vi "Gel Tugging Force Mode_Data Reduction v16.00.vi"() -> ()   [LabVIEW 2015]
doc: "I. Description:\nThis example demonstrates how to continuously acquire and generate data at the same time, synchronized with one another.\n\nII. Instructions for Running:\n1. Select the physical channel to correspond to where your signal is input on the DAQ device. Also, select the corresponding channel for where your signal is being generated.\n2. Enter the minimum and maximum voltage ranges.\nNote: For better accuracy try to match the input range to the expected voltage level of the measured signal.\n3. Set the sample rate of the acquisition.\nNote: The rate should be at least twice as fast as the maximum frequency component of the signal being acquired. \n6. Select the Rate for the generation\n7. Select what type of signal to generate and the amplitude.\nNote: This example requires two DMA channels to run. If your hardware does not support two DMA channels, you need to set the Data Transfer Mechanism property for the Analog Output Task to use \"Interrupts\". The Data Transfer Mechanism property is located in the DAQmx Channel Property hierarchy at:\n\nDAQmx Channel Property Node>>Analog Output>>General Properties>>Advanced>>Data Transfer and Memory>>Data Transfer Mechanism\n\nRefer to your device documentation to determine how many DMA channels are supported for your hardware.\n\nIII. Block Diagram Steps:\n1. Create an analog input voltage channel. Also, create an analog output voltage channel.\n2. Set the rate for the sample clock. Additionally, define the sample mode to be continuous. Also, set the sample clock rate for the signal generation.\n2a. Call the Get Terminal Name with Device Prefix VI. This will take a Task and a terminal and create a properly formatted device + terminal name to use as the source of the Trigger.\n3. Define the parameters for a Digital Edge Start Trigger. Set the Analog output to trigger off the AI Start Trigger. This is an internal trigger signal.\n4. Use the Basic Function Generator VI to create the signal to be generated.\n5. Call the Start VI to arm the two functions. Make sure the analog output is armed before the analog input. This will ensure both will start at the same time.\n6. Read the waveform data in a loop until the user hits the stop button or an error occurs. The Is Task Done? VI is used to check for errors in the Analog Output Task.\n7. Call the Clear VI to Clear the Task\n8. Use the popup dialog box to display an error if any.\n\nIV. I/O Connections Overview:\nMake sure your signal input/output terminals match the Physical Channel I/O controls."
uses:
  <vilib>/Utility/file.llb/Read Delimited Spreadsheet (DBL).vi
  <vilib>/Analysis/NI_AALBase.lvlib
  <vilib>/Analysis/NI_AALPro.lvlib
panel:
  out "Total Ramp\n Time (ms)":dbl format="%#_10g"
  out "# of Ramp\n Steps":dbl format="%#_10g"
  out "Fluoro Bead \nDiameter (um)":dbl format="%#_10g"
  out "Image Scale (Micron/Pixel)":dbl format="%#_10g"
  out "Initial Sep Distance (Micron)":dbl format="%#_10g"
  out "Fluoro Beads Z-Level (micron)":dbl format="%#_10g"
  out "Gel Thickness (micron)":dbl format="%#_10g"
  out "Magnetic Bead Z-Level (micron)":dbl format="%#_10g"
  out "Tip Z-Level (micron)":dbl format="%#_10g"
  out "Exposure \nPulses":i32
  out "Magnetic Bead Diameter (um)":dbl format="%#_10g"
  out "Null Flux\nCorrected (Gs)":dbl format="%#_10g"
  out "95% C.I. Maximum":dbl format="%_8f"
  out "95% C.I. Minimum":dbl format="%_8f"
  out "Current, Std Dev (V or Amp)":dbl format="%_8g"
  out "Current, Mean (V or Amp) 2":dbl format="%_8g"
  out "Slope of Trendline \n(mV of mAmp/min)":dbl
  out "Slope of Trendline \n(V or Amp/sec)":dbl
  out "Intercept of Trendline (V or Amp)":dbl format="%#_8g"
  out "Slope of Trendline \n(mV of mAmp/min)":dbl
  out "Intercept of Trendline (V or Amp)":dbl format="%#_8g"
  out "Slope of Trendline \n(V or Amp/sec)":dbl
  out "95% C.I. Maximum":dbl format="%_8f"
  out "95% C.I. Minimum":dbl format="%_8f"
  out "Current, Std Dev (V or Amp)":dbl format="%_8g"
  out "Current, Mean (V or Amp)":dbl format="%_8g"
  in  "Final Time 2 (s)":dbl=3.0 format="%_8g"
  in  "Initial Time 2 (s)":dbl=2.05 format="%_8g"
  out "Current Signal (V)":cluster{dbl[], dbl[]}(graph)
  out "Slope of Trendline \n(mGs/min)":dbl
  out "Intercept of Trendline (Gs)":dbl format="%#_8g"
  out "Slope of Trendline \n(Gs/sec)":dbl
  out "95% C.I. Maximum":dbl format="%_8f"
  out "95% C.I. Minimum":dbl format="%_8f"
  out "Magnetic Flux, Std Dev (Gs)":dbl format="%_8g"
  out "Magnetic Flux, Mean (Gs)":dbl format="%_8g"
  out "OFF PID gains":T1={"proportional gain (Kc)"=0.8, "integral time (Ti, min)"=3e-05, "derivative time (Td, min)"=4.7e-06} {"proportional gain (Kc)" format="%#_10g"; "integral time (Ti, min)" format="%#_10g"; "derivative time (Td, min)" format="%#_10g"}
  out "Relative Humidity (%)":dbl format="%#_10g"
  out "Needle Inclination Angle (º)":dbl format="%#_10g"
  out "Temperature (ºC)":dbl format="%#_10g"
  out "Post- Zero\nInterval (s) <(If not  interrupted)":dbl format="%#_10g"
  out "Pre- Zero \nInterval (s)":dbl format="%#_10g"
  out "Null Flux\nObserved (Gs)":dbl format="%#_10g"
  out "Flux ON Relative \nSetpoint (Gs)":dbl format="%#_10g"
  in  "Final Time 1 (s)":dbl=2.0 format="%_8g"
  in  "Initial Time 1 (s)":dbl=1.05 format="%_8g"
  out "PID Rate (Hz)":dbl format="%#_10g"
  out "Sampling Rate \n(Samples/Sec)":dbl format="%#_10g"
  out "ON PID gains":T1={"proportional gain (Kc)"=0.8, "integral time (Ti, min)"=3e-05, "derivative time (Td, min)"=4.7e-06} {"proportional gain (Kc)" format="%#_10g"; "integral time (Ti, min)" format="%#_10g"; "derivative time (Td, min)" format="%#_10g"}
  out "Samples Pushed \nto PID at a time":dbl format="%#_10g"
  out "Camera Exposure (V)":cluster{dbl[], dbl[]}(graph)
  out "# of Data Points":i32
  out "Sampling\nInterval (ms)":dbl format="%#_8g"
  out "Slope of Trendline \n(mGs/min)":dbl
  out "Intercept of Trendline (V)":dbl format="%#_8g"
  out "Slope of Trendline \n(Gs/sec)":dbl
  out "95% C.I. Maximum":dbl format="%_8f"
  out "95% C.I. Minimum":dbl format="%_8f"
  out "Magnetic Flux, Std Dev (Gs)":dbl format="%_8g"
  out "Magnetic Flux, Mean (Gs)":dbl format="%_8g"
  out "Magnetic Sensor \nSensitivity (V/Gs)":dbl
  out "Flux Signal, V":cluster{dbl[], dbl[]}(graph)
  out "Magnetic Sensor \nCalibrated Zero (V)":dbl format="%#_12g"
  out "Number of \nCycles":dbl format="%#_10g"
  out "Flux Signal, Gs":cluster{dbl[], dbl[]}(graph)
  in  "Select data file for reduction...":path
  # "Gel Testing v.15.00 + v15.10 + v15.20"
  # "Drift Analysis For Flux & Current:"
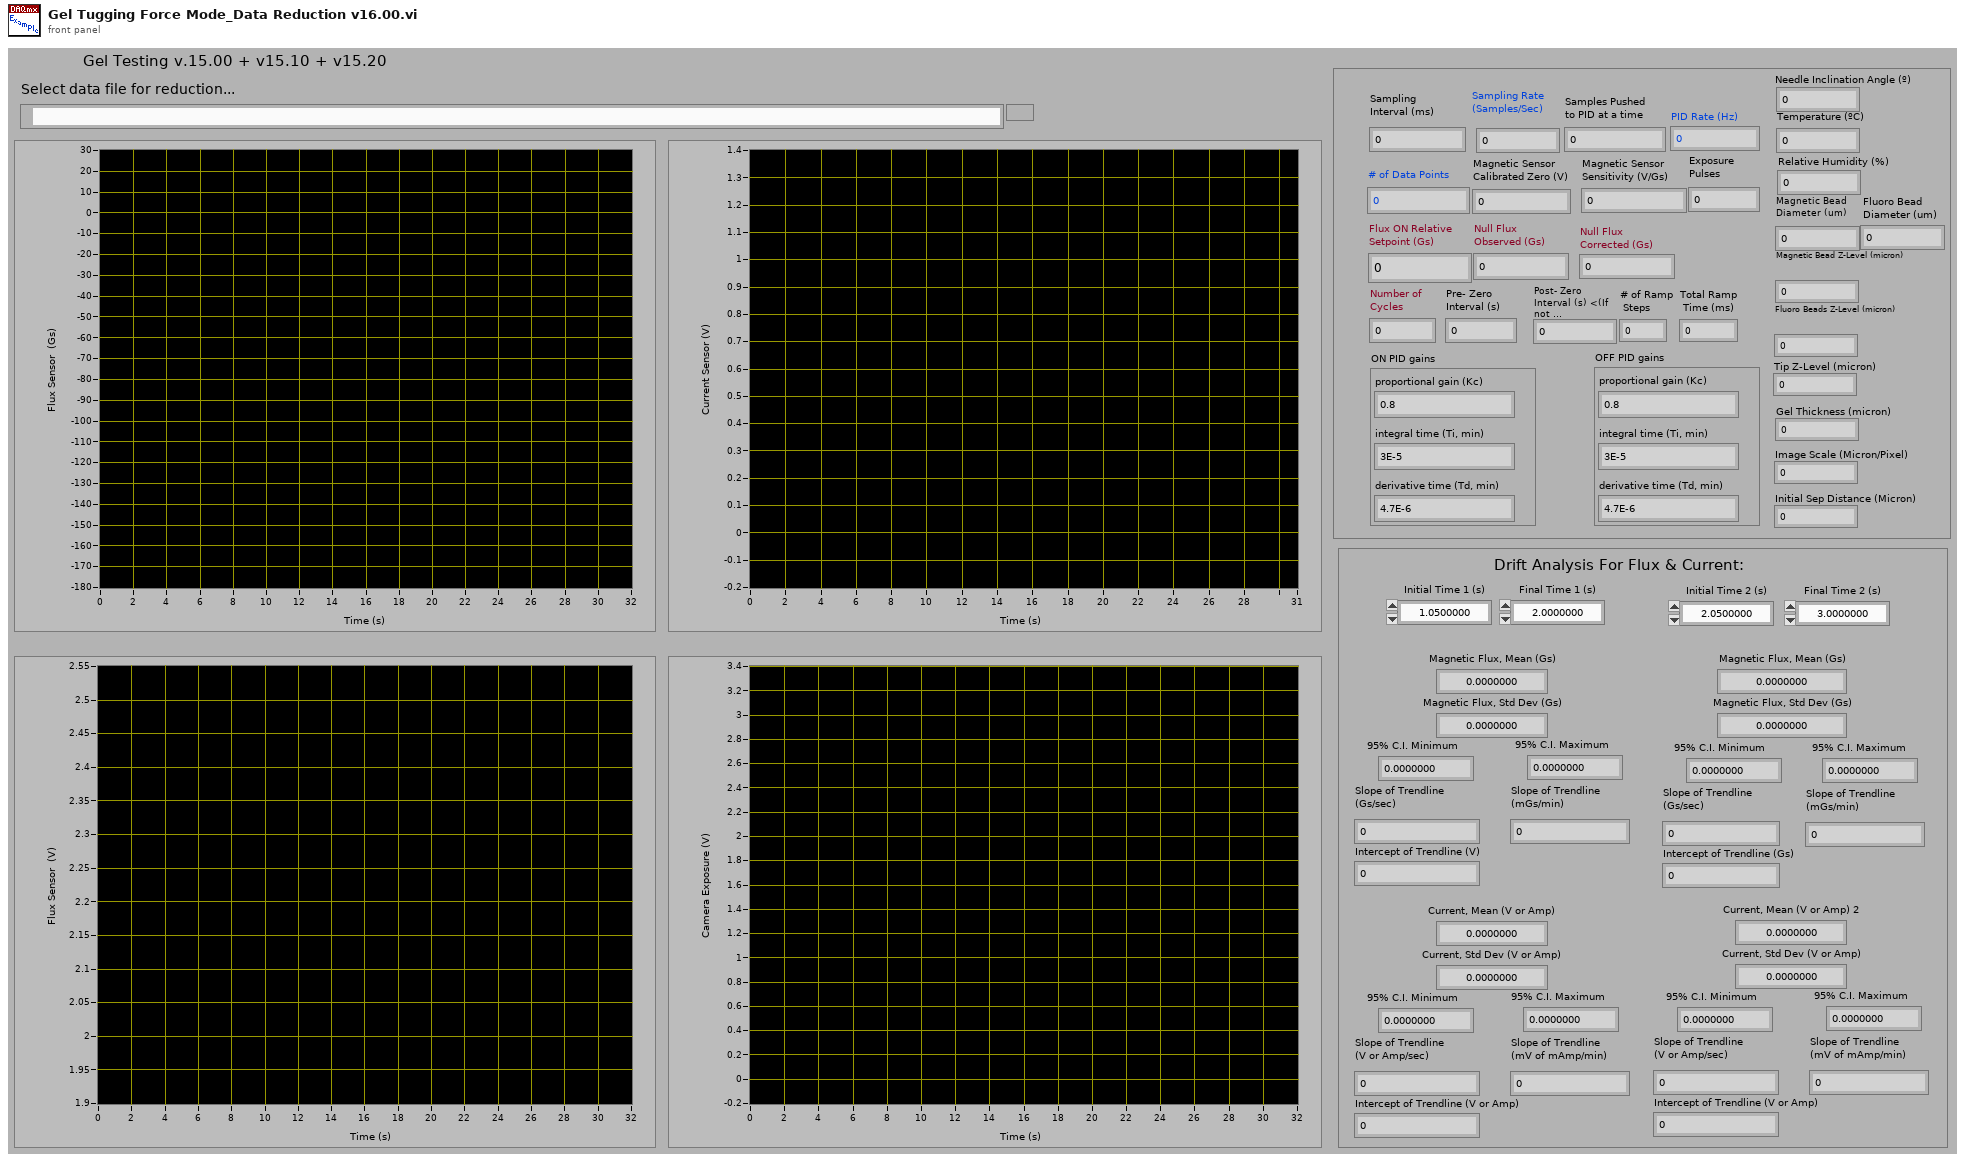
[diagram p1: front panel]
types:
  T1 = cluster{"proportional gain (Kc)":dbl, "integral time (Ti, min)":dbl, "derivative time (Td, min)":dbl}
  T2 = cluster{"Numeric":dbl, "Numeric":dbl, "Numeric":dbl}
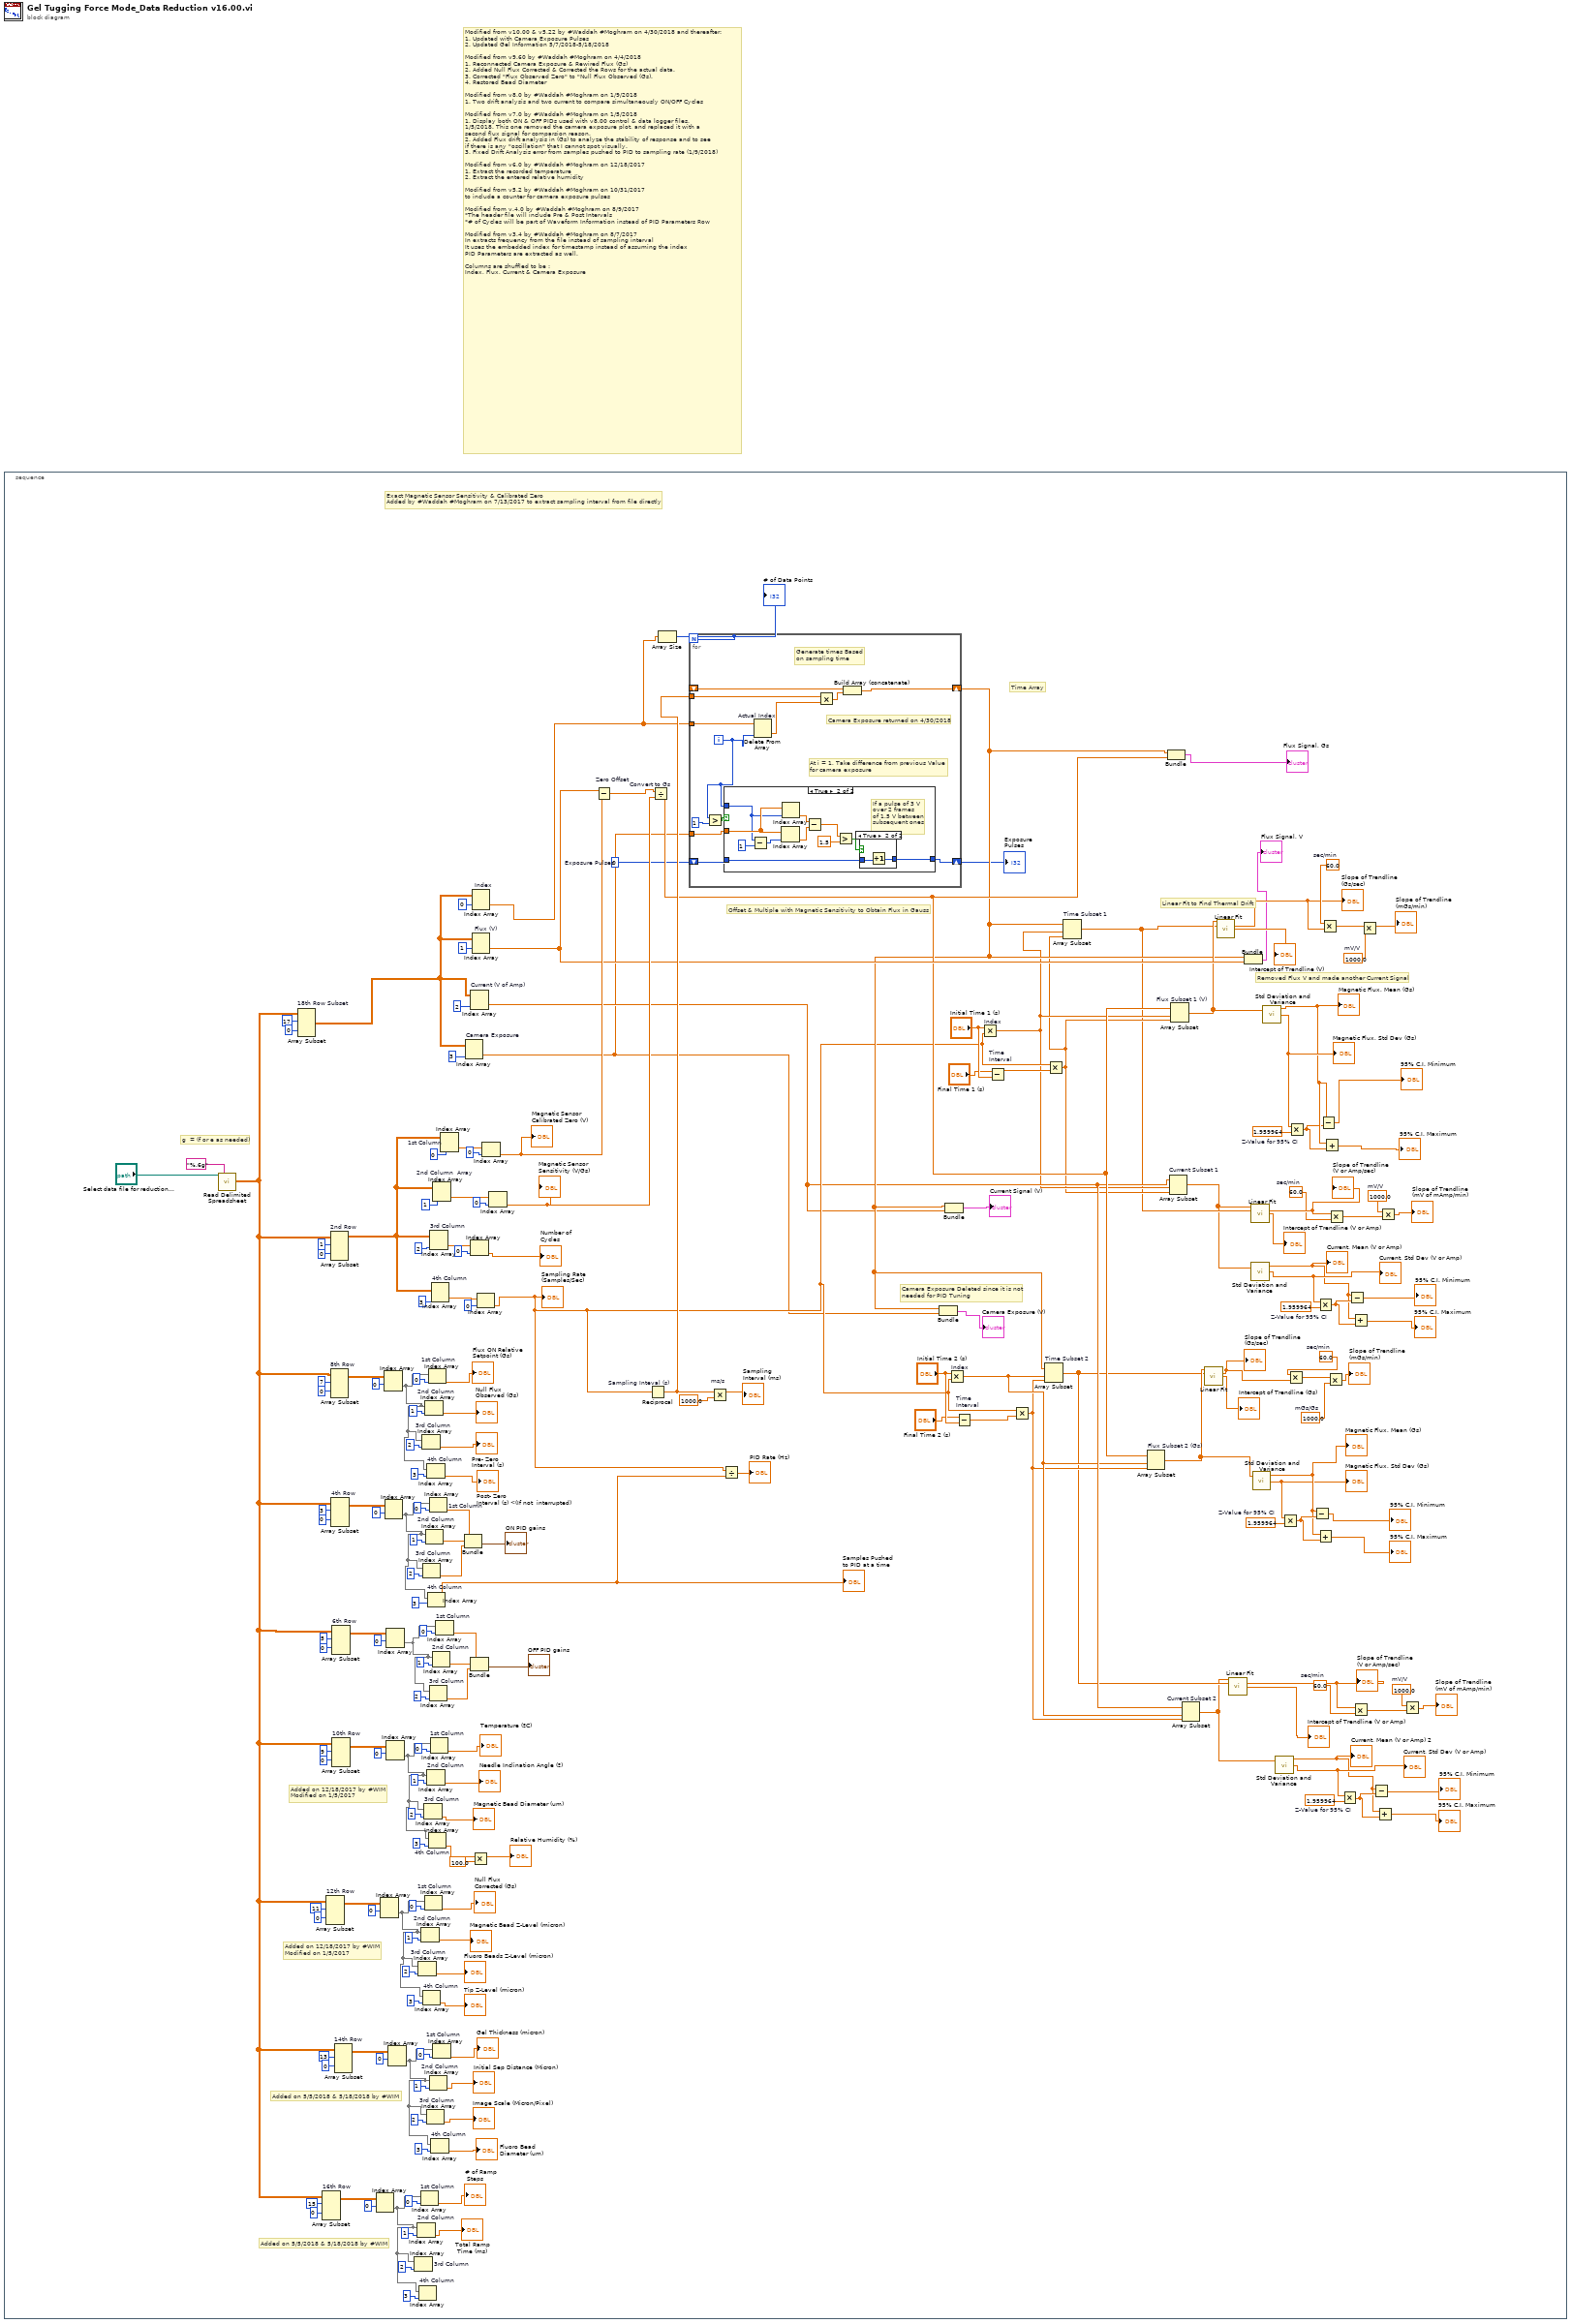
[diagram p0: block diagram]
diagram:
  # "Modified from v10.00 & v5.22 by #Waddah #Moghram on 4/30/2018 and thereafter: \n1. Updated with Camera Exposure Pulses\n2. Updated Gel Information 5/7/2018-5/18/2018\n\nModified from v9.60 by #Waddah #Moghram on 4/4/2018\n1. Reconnected Camera Exposure & Rewired Flux (Gs)\n2. Added Null Flux Corrected & Corrected the Rows for the actual data.\n3. Corrected \"Flux Observed Zero\" to \"Null Flux Observed (Gs). \n4. Restored Bead Diameter\n\nModified from v8.0 by #Waddah #Moghram on 1/9/2018\n1. Two drift analysis and two current to compare simultaneously ON/OFF Cycles\n\nModified from v7.0 by #Waddah #Moghram on 1/5/2018\n1. Display both ON & OFF PIDs used with v8.00 control & data logger files.\n1/5/2018. This one removed the camera exposure plot, and replaced it with a \nsecond flux signal for comparsion reason.\n2. Added Flux drift analysis in (Gs) to analyze the stability of response and to see\nif there is any \"oscillation\" that I cannot spot visually.\n3. Fixed Drift Analysis error from samples pushed to PID to sampling rate (1/9/2018)\n\nModified from v6.0 by #Waddah #Moghram on 12/18/2017\n1. Extract the recorded temperature\n2. Extract the entered relative humidity\n\nModified from v5.2 by #Waddah #Moghram on 10/31/2017 \nto include a counter for camera exposure pulses\n\nModified from v.4.0 by #Waddah #Moghram on 8/9/2017\n*The header file will include Pre & Post Intervals\n*# of Cycles will be part of Waveform Information instead of PID Parameters Row\n\nModified from v3.4 by #Waddah #Moghram on 8/7/2017\nIn extracts frequency from the file instead of sampling interval \nIt uses the embedded index for timestamp instead of assuming the index\nPID Parameters are extracted as well.\n\nColumns are shuffled to be :\nIndex, Flux, Current & Camera Exposure"
  n1 = stacked-sequence {
    frame #0 {
      w30 = 0  # Exposure Pulses
      w55 = 1.959964  # Z-Value for 95% CI
      w57 = 1000.0  # mV/V
      w59 = 60.0  # sec/min
      w64 = 1.959964  # Z-Value for 95% CI
      w67 = 1000.0  # mV/V
      w69 = 60.0  # sec/min
      w92 = 60.0  # sec/min
      w93 = 1000.0  # mGs/Gs
      w100 = 1.959964  # Z-Value for 95% CI
      w166 = 1000.0  # mV/V
      w169 = 60.0  # sec/min
      w177 = 1.959964  # Z-Value for 95% CI
      # "Added on 5/5/2018 & 5/18/2018 by #WIM"
      # "Added on 5/5/2018 & 5/18/2018 by #WIM"
      # "Added on 12/18/2017 by #WIM\nModified on 1/5/2017"
      # "Time Array"
      # "Removed Flux V and made another Current Signal"
      # "Camera Exposure Deleted since it is not \nneeded for PID Tuning"
      # "Added on 12/18/2017 by #WIM\nModified on 1/5/2017"
      # "g  = (f or e as needed)"
      # "Linear Fit to Find Thermal Drift"
      # "Offset & Multiple with Magnetic Sensitivity to Obtain Flux in Gauss"
      # "Exact Magnetic Sensor Sensitivity & Calibrated Zero\nAdded by #Waddah #Moghram on 7/13/2017 to extract sampling interval from file directly"
      n2 = call-poly <vilib>:"Read Delimited Spreadsheet.vi"("file path (dialog if empty)"="Select data file for reduction...", "format (%.3f)"="%.6g") -> ("all rows"=w4:dbl[][])  [unwired: 8 in, 5 out]
      n3 = Array Subset "18th Row Subset"(array=w4, index (row)=17 ("index"), index (col)=0 ("index")) -> (w162:dbl[][])  [unwired: 2 in]
      n4 = Array Subset "16th Row"(array=w4, index (row)=15 ("index"), index (col)=0 ("index")) -> (w9:dbl[][])  [unwired: 2 in]
      n5 = Array Subset "12th Row"(array=w4, index (row)=11 ("index"), index (col)=0 ("index")) -> (w38:dbl[][])  [unwired: 2 in]
      n6 = Array Subset "2nd Row"(array=w4, index (row)=1 ("index"), index (col)=0 ("index")) -> (w180:dbl[][])  [unwired: 2 in]
      n7 = Array Subset "8th Row"(array=w4, index (row)=7 ("index"), index (col)=0 ("index")) -> (w135:dbl[][])  [unwired: 2 in]
      n8 = Array Subset "4th Row"(array=w4, index (row)=3 ("index"), index (col)=0 ("index")) -> (w150:dbl[][])  [unwired: 2 in]
      n9 = Array Subset "6th Row"(array=w4, index (row)=5 ("index"), index (col)=0 ("index")) -> (w103:dbl[][])  [unwired: 2 in]
      n10 = Array Subset "10th Row"(array=w4, index (row)=9 ("index"), index (col)=0 ("index")) -> (w120:dbl[][])  [unwired: 2 in]
      n11 = Array Subset "14th Row"(array=w4, index (row)=13 ("index"), index (col)=0 ("index")) -> (w22:dbl[][])  [unwired: 2 in]
      n12 = Index Array(array=w9, index (row)=0) -> (element=w7:dbl[])  [unwired: 1 in]
      n13 = Index Array(array=w38, index (row)=0) -> (element=w36:dbl[])  [unwired: 1 in]
      n14 = Index Array(array=w135, index (row)=0) -> (element=w133:dbl[])  [unwired: 1 in]
      n15 = Index Array(array=w150, index (row)=0) -> (element=w148:dbl[])  [unwired: 1 in]
      n16 = Index Array(array=w103, index (row)=0) -> (element=w102:dbl[])  [unwired: 1 in]
      n17 = Index Array(array=w120, index (row)=0) -> (element=w118:dbl[])  [unwired: 1 in]
      n18 = Index Array(array=w22, index (row)=0) -> (element=w20:dbl[])  [unwired: 1 in]
      n19 = Index Array "3rd Column"(array=w7, index=2) -> ()  [unwired: 1 out]
      n20 = Index Array "2nd Column"(array=w7, index=1) -> (element=→"Total Ramp\n Time (ms)":dbl)
      n21 = Index Array "3rd Column"(array=w36, index=2) -> (element=→"Fluoro Beads Z-Level (micron)":dbl)
      n22 = Index Array "4th Column"(array=w7, index=3) -> ()  [unwired: 1 out]
      n23 = Index Array "1st Column"(array=w7, index=0) -> (element=→"# of Ramp\n Steps":dbl)
      n24 = Index Array "2nd Column"(array=w36, index=1) -> (element=→"Magnetic Bead Z-Level (micron)":dbl)
      n25 = Index Array "3rd Column"(array=w133, index=2) -> (element=→"Pre- Zero \nInterval (s)":dbl)
      n26 = Index Array "3rd Column"(array=w148, index=2) -> (element=w151:dbl)
      n27 = Index Array "4th Column"(array=w36, index=3) -> (element=→"Tip Z-Level (micron)":dbl)
      n28 = Index Array "3rd Column"(array=w118, index=2) -> (element=→"Magnetic Bead Diameter (um)":dbl)
      n29 = Index Array "1st Column"(array=w36, index=0) -> (element=→"Null Flux\nCorrected (Gs)":dbl)
      n30 = Index Array "2nd Column"(array=w133, index=1) -> (element=→"Null Flux\nObserved (Gs)":dbl)
      n31 = Index Array "2nd Column"(array=w148, index=1) -> (element=w152:dbl)
      n32 = Index Array "3rd Column"(array=w20, index=2) -> (element=→"Image Scale (Micron/Pixel)":dbl)
      n33 = Index Array "4th Column"(array=w133, index=3) -> (element=→"Post- Zero\nInterval (s) <(If not  interrupted)":dbl)
      n34 = Index Array "2nd Column"(array=w118, index=1) -> (element=→"Needle Inclination Angle (º)":dbl)
      n35 = Index Array "4th Column"(array=w148, index=3) -> (element=w87:dbl)
      "Samples Pushed \nto PID at a time" <- w87
      n36 = Index Array "1st Column"(array=w133, index=0) -> (element=→"Flux ON Relative \nSetpoint (Gs)":dbl)
      n37 = Index Array "4th Column"(array=w118, index=3) -> (element=w115:dbl)
      n38 = Index Array "1st Column"(array=w148, index=0) -> (element=w153:dbl)
      n39 = Index Array "3rd Column"(array=w102, index=2) -> (element=w104:dbl)
      n40 = Index Array "2nd Column"(array=w20, index=1) -> (element=→"Initial Sep Distance (Micron)":dbl)
      n41 = Index Array "3rd Column"(array=w180, index (col)=2) -> (element=w193:dbl[])  [unwired: 1 in]
      n42 = Index Array "1st Column"(array=w118, index=0) -> (element=→"Temperature (ºC)":dbl)
      n43 = Index Array "4th Column"(array=w20, index=3) -> (element=→"Fluoro Bead \nDiameter (um)":dbl)
      n44 = Index Array "4th Column"(array=w180, index (col)=3) -> (element=w190:dbl[])  [unwired: 1 in]
      n45 = Index Array "2nd Column"(array=w102, index=1) -> (element=w105:dbl)
      n46 = Index Array "2nd Column  Array"(array=w180, index (col)=1) -> (element=w182:dbl[])  [unwired: 1 in]
      n47 = Index Array "1st Column"(array=w20, index=0) -> (element=→"Gel Thickness (micron)":dbl)
      n48 = Index Array "1st Column"(array=w102, index=0) -> (element=w106:dbl)
      n49 = Index Array "1st Column"(array=w180, index (col)=0) -> (element=w186:dbl[])  [unwired: 1 in]
      n50 = Bundle("Numeric"=w153, "Numeric"=w152, "Numeric"=w151) -> (→"ON PID gains":T2)  [unwired: 1 in]
      n51 = Index Array "Camera Exposure"(array=w162, index (col)=3) -> (element=w31:dbl[])  [unwired: 1 in]
      n52 = Index Array "Current (V of Amp)"(array=w162, index (col)=2) -> (element=w78:dbl[])  [unwired: 1 in]
      n53 = Index Array(array=w193, index=0) -> (element=→"Number of \nCycles":dbl)
      n54 = Bundle("Numeric"=w106, "Numeric"=w105, "Numeric"=w104) -> (→"OFF PID gains":T2)  [unwired: 1 in]
      n55 = Multiply(x=w115, y=100.0) -> (x*y=→"Relative Humidity (%)":dbl)
      n56 = Index Array "Index"(array=w162, index (col)=0) -> (element=w161:dbl[])  [unwired: 1 in]
      n57 = Index Array "Flux (V)"(array=w162, index (col)=1) -> (element=w143:dbl[])  [unwired: 1 in]
      n58 = Index Array(array=w190, index=0) -> (element=w79:dbl)
      "Sampling Rate \n(Samples/Sec)" <- w79
      n59 = Index Array(array=w186, index=0) -> (element=w147:dbl)
      "Magnetic Sensor \nCalibrated Zero (V)" <- w147
      n60 = Index Array(array=w182, index=0) -> (element=w178:dbl)
      "Magnetic Sensor \nSensitivity (V/Gs)" <- w178
      n61 = Subtract "Zero Offset"(x=w143, y=w147) -> (x-y=w179:dbl[])
      n62 = Reciprocal "Sampling Inteval (s)"(x=w79) -> (1/x=w164:dbl)
      n63 = Divide "Convert to Gs"(x=w179, y=w178) -> (x/y=w81:dbl[])
      n64 = Array Size(array=w161) -> (size(s)=w188:i32)
      "# of Data Points" <- w188
      n65 = for {
        N: w188 -> [_]
        shift-right: [w214] -> w80
        shift-left: _ -> [w213]
        tunnel: w164 -> [w211]
        tunnel: w161 -> [w210]
        tunnel: w31 -> [w205]
        shift-right: [w203] -> w29
        shift-left: w30 -> [w204]
        i -> [w206]
        # "Camera Exposure returned on 4/30/2018"
        # "At i = 1, Take difference from previous Value \nfor camera exposure"
        # "Generate times Based \non sampling time"
        n66 = Greater?(x=w206, y=1) -> (0:w207:bool)
        n67 = case shown="True" w207 {
          tunnel: w205 -> [_ w226]
          tunnel: w206 -> [_ w224]
          tunnel: w204 -> [w215 w220]
          tunnel: [w215 w219] -> w203
          frame False {
          }
          frame True {
            # "If a pulse of 3 V\nover 2 frames \nof 1.5 V between\nsubsequent ones"
            n68 = Subtract(x=w224, y=1) -> (x-y=w225:i32)
            n69 = Index Array(array=w226, index=w225) -> (element=w221:dbl)
            n70 = Index Array(array=w226, index=w224) -> (element=w222:dbl)
            n71 = Subtract(x=w222, y=w221) -> (x-y=w218:dbl)
            n72 = Greater?(x=w218, y=1.5) -> (0:w216:bool)
            n73 = case shown="True" w216 {
              tunnel: w220 -> [w227 w229]
              tunnel: [w227 w228] -> w219
              frame False {
              }
              frame True {
                n74 = Increment(x=w229) -> (x+1=w228:i32)
              }
            }
          }
        }
        n75 = Delete From Array "Actual Index"(array=w210, index=w206) -> (deleted portion=w209:dbl)  [unwired: 1 in, 1 out]
        n76 = Multiply(x=w211, y=w209) -> (x*y=w212:dbl)
        n77 = Build Array (concatenate)(w213, w212) -> (w214:dbl[])
      }
      "Exposure \nPulses" <- w29
      n78 = Multiply "ms/s"(x=w164, y=1000.0) -> (x*y=→"Sampling\nInterval (ms)":dbl)
      n79 = Divide(x=w79, y=w87) -> (x/y=→"PID Rate (Hz)":dbl)
      n80 = Bundle(w80, w31) -> (→"Camera Exposure (V)":cluster{dbl[], dbl[]})  [unwired: 1 in]
      n81 = Bundle(w80, w78) -> (→"Current Signal (V)":cluster{dbl[], dbl[]})  [unwired: 1 in]
      n82 = Multiply "Index"(x="Initial Time 2 (s)", y=w79) -> (x*y=w75:dbl)
      n83 = Subtract "Time\nInterval"(x="Final Time 2 (s)", y="Initial Time 2 (s)") -> (x-y=w82:dbl)
      n84 = Multiply "Index"(x="Initial Time 1 (s)", y=w79) -> (x*y=w77:dbl)
      n85 = Subtract "Time\nInterval"(x="Final Time 1 (s)", y="Initial Time 1 (s)") -> (x-y=w86:dbl)
      n86 = Multiply(x=w79, y=w82) -> (x*y=w74:dbl)
      n87 = Array Subset "Time Subset 2"(array=w80, index=w75, length=w74) -> (w72:dbl[])
      n88 = Multiply(x=w79, y=w86) -> (x*y=w76:dbl)
      n89 = Array Subset "Time Subset 1"(array=w80, index=w77, length=w76) -> (w73:dbl[])
      n90 = Array Subset "Flux Subset 2 (Gs)"(array=w81, index=w75, length=w74) -> (w89:dbl[])
      n91 = Bundle(w80, w81) -> (→"Flux Signal, Gs":cluster{dbl[], dbl[]})  [unwired: 1 in]
      n92 = Array Subset "Current Subset 1"(array=w78, index=w77, length=w76) -> (w65:dbl[])
      n93 = Array Subset "Flux Subset 1 (V)"(array=w81, index=w77, length=w76) -> (w142:dbl[])
      n94 = Array Subset "Current Subset 2"(array=w78, index=w75, length=w74) -> (w48:dbl[])
      n95 = call <vilib>:"Linear Fit.vi"("Y"=w89, "X"=w72) -> ("slope"=w91:dbl, "intercept"=→"Intercept of Trendline (Gs)":dbl)  [unwired: 9 in, 3 out]
      "Slope of Trendline \n(Gs/sec)" <- w91
      n96 = call <vilib>:"Linear Fit.vi"("Y"=w142, "X"=w73) -> ("slope"=w168:dbl, "intercept"=→"Intercept of Trendline (V)":dbl)  [unwired: 9 in, 3 out]
      "Slope of Trendline \n(Gs/sec)" <- w168
      n97 = call <vilib>:"Linear Fit.vi"("Y"=w48, "X"=w72) -> ("slope"=w50:dbl, "intercept"=→"Intercept of Trendline (V or Amp)":dbl)  [unwired: 9 in, 3 out]
      "Slope of Trendline \n(V or Amp/sec)" <- w50
      n98 = Bundle(w80, w143) -> (→"Flux Signal, V":cluster{dbl[], dbl[]})  [unwired: 1 in]
      n99 = call <vilib>:"Linear Fit.vi"("Y"=w65, "X"=w73) -> ("slope"=w70:dbl, "intercept"=→"Intercept of Trendline (V or Amp)":dbl)  [unwired: 9 in, 3 out]
      "Slope of Trendline \n(V or Amp/sec)" <- w70
      n100 = call <vilib>:"Std Deviation and Variance.vi"("X"=w65) -> ("mean"=w47:dbl, "standard deviation"=w62:dbl)  [unwired: 1 in, 1 out]
      "Current, Mean (V or Amp)" <- w47
      "Current, Std Dev (V or Amp)" <- w62
      n101 = call <vilib>:"Std Deviation and Variance.vi"("X"=w89) -> ("mean"=w98:dbl, "standard deviation"=w88:dbl)  [unwired: 1 in, 1 out]
      "Magnetic Flux, Mean (Gs)" <- w98
      "Magnetic Flux, Std Dev (Gs)" <- w88
      n102 = call <vilib>:"Std Deviation and Variance.vi"("X"=w142) -> ("mean"=w175:dbl, "standard deviation"=w176:dbl)  [unwired: 1 in, 1 out]
      "Magnetic Flux, Mean (Gs)" <- w175
      "Magnetic Flux, Std Dev (Gs)" <- w176
      n103 = call <vilib>:"Std Deviation and Variance.vi"("X"=w48) -> ("mean"=w46:dbl, "standard deviation"=w53:dbl)  [unwired: 1 in, 1 out]
      "Current, Mean (V or Amp) 2" <- w46
      "Current, Std Dev (V or Amp)" <- w53
      n104 = Multiply(x=w88, y=w100) -> (x*y=w99:dbl)
      n105 = Multiply(x=w92, y=w91) -> (x*y=w95:dbl)
      n106 = Multiply(x=w176, y=w177) -> (x*y=w172:dbl)
      n107 = Subtract(x=w98, y=w99) -> (x-y=→"95% C.I. Minimum":dbl)
      n108 = Multiply(x=w62, y=w64) -> (x*y=w63:dbl)
      n109 = Add(x=w98, y=w99) -> (x+y=→"95% C.I. Maximum":dbl)
      n110 = Subtract(x=w175, y=w172) -> (x-y=→"95% C.I. Minimum":dbl)
      n111 = Multiply(x=w169, y=w168) -> (x*y=w170:dbl)
      n112 = Add(x=w175, y=w172) -> (x+y=→"95% C.I. Maximum":dbl)
      n113 = Multiply(x=w95, y=w93) -> (x*y=→"Slope of Trendline \n(mGs/min)":dbl)
      n114 = Multiply(x=w70, y=w69) -> (x*y=w68:dbl)
      n115 = Multiply(x=w53, y=w55) -> (x*y=w54:dbl)
      n116 = Subtract(x=w47, y=w63) -> (x-y=→"95% C.I. Minimum":dbl)
      n117 = Add(x=w47, y=w63) -> (x+y=→"95% C.I. Maximum":dbl)
      n118 = Multiply(x=w50, y=w59) -> (x*y=w58:dbl)
      n119 = Multiply(x=w170, y=w166) -> (x*y=→"Slope of Trendline \n(mGs/min)":dbl)
      n120 = Subtract(x=w46, y=w54) -> (x-y=→"95% C.I. Minimum":dbl)
      n121 = Add(x=w46, y=w54) -> (x+y=→"95% C.I. Maximum":dbl)
      n122 = Multiply(x=w67, y=w68) -> (x*y=→"Slope of Trendline \n(mV of mAmp/min)":dbl)
      n123 = Multiply(x=w57, y=w58) -> (x*y=→"Slope of Trendline \n(mV of mAmp/min)":dbl)
    }
  }
